vi "close.vi"(8 "error in":errorcluster, 11 "tag bus configurable plugin module in":refnum<class "tag bus configurable plugin module.lvclass">) -> (0 "error out":errorcluster)   [LabVIEW 2013, in "tag bus configurable plugin module.lvclass"]
doc: "Provides an interface for terminating a module instance. While this interface performs no operations, a child should close and deallocate any open references or memory."
uses:
  tag bus configurable plugin module.lvclass
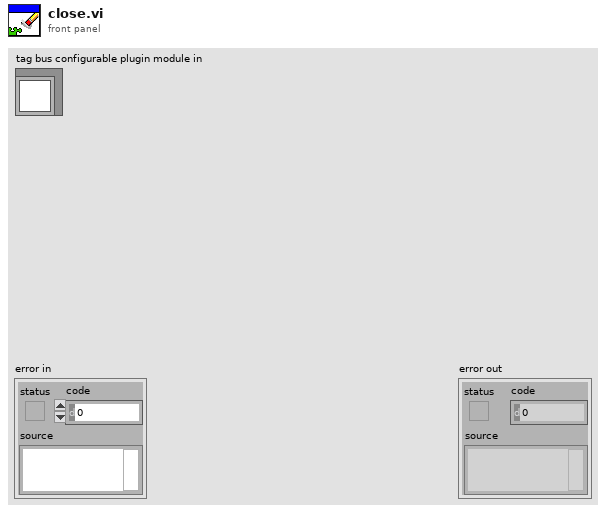
[diagram p1: front panel]
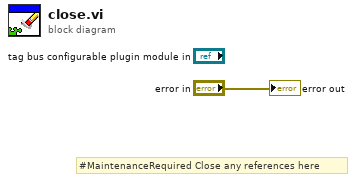
[diagram p0: block diagram]
diagram:
  # "#MaintenanceRequired Close any references here"
  "error out" <- "error in"
